vi "Replication and Deployment Utility.vi"() -> ()   [LabVIEW 2016]
uses:
  subVIs/TypeDefs/rad_State Data.ctl
  subVIs/Targets/TypeDefs/rad_Targets Settings.ctl
  subVIs/Targets/TypeDefs/rad_Target Information.ctl
  subVIs/Targets/TypeDefs/rad_Target Network Settings.ctl
  subVIs/App Images/TypeDefs/rad_App Images Settings.ctl
  subVIs/App Images/TypeDefs/rad_AppImage Information.ctl
  subVIs/App Images/TypeDefs/rad_Application Image Properties.ctl
  subVIs/App Images/TypeDefs/rad_FPGA Properties.ctl
  subVIs/App Images/TypeDefs/rad_FPGA Flash Properties.ctl
  subVIs/Util/Controls/Exit Button.ctl
  subVIs/Util/Controls/Retrieve Button.ctl
  subVIs/Util/Controls/Refresh Button.ctl
  subVIs/Util/Controls/Configure Button.ctl
  subVIs/Util/Controls/Deploy Button.ctl
  subVIs/Util/Controls/Select All Button.ctl
  subVIs/Util/Controls/Add Target Button.ctl
  subVIs/Util/Controls/Compare Button.ctl
  subVIs/Util/FP Control/FP Control Functions.ctl
  <vilib>/Utility/miscctls.llb/LVRowAndColumnUnsignedTypeDef.ctl
  subVIs/RT Image Compare/TypeDefs/rad_Comparison Modes.ctl
  subVIs/rad_Globals.vi
  <vilib>/nisyscfg/Close (System).vi
  <vilib>/nisyscfg/nisyscfg.lvlib
  <resource>/objmgr/nisysapi.rc
panel:
  in  "Targets Settings":bool
  in  "Refresh Targets":T1
  in  "Target List":i32[](listbox)=[0]
  in  "Add Target":T2
  in  "Select All":T3
  in  "Configure Targets":T4
  in  "Compare":T5
  in  "Deploy":T6
  in  "Retrieve":T7
  in  "State":T8 {"Targets Information"."Primary NIC"."IP Address Request Mode" items=["Static"=1, "DHCP/Link-Local"=2, "Link-Local Only"=4, "DHCP Only"=8]}
  in  "App Images Settings":bool
  in  "Refresh Apps":T1
  in  "Exit":T17
  in  "App Images List":i32(listbox)=6
  in  "Configure App":T4
  # "Deployment Targets"
  # "Application Images"
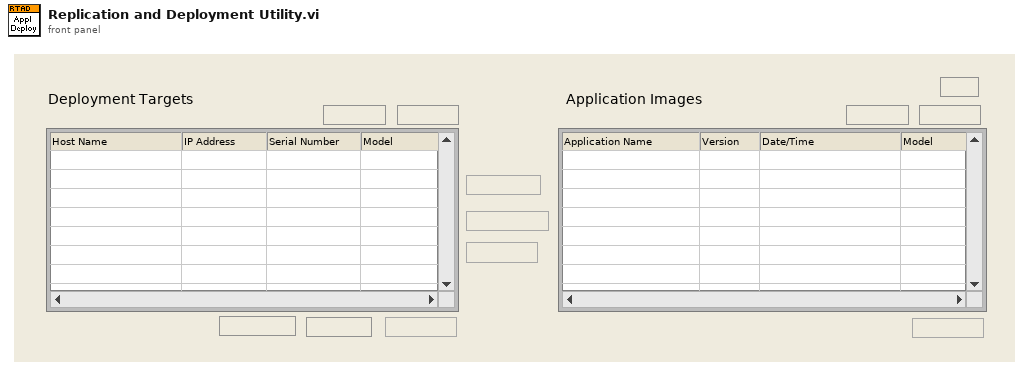
[diagram p1: front panel]
types:
  T1 = typedef "Refresh Button.ctl" = bool
  T2 = typedef "Add Target Button.ctl" = bool
  T3 = typedef "Select All Button.ctl" = bool
  T4 = typedef "Configure Button.ctl" = bool
  T5 = typedef "Compare Button.ctl" = bool
  T6 = typedef "Deploy Button.ctl" = bool
  T7 = typedef "Retrieve Button.ctl" = bool
  T8 = typedef "rad_State Data.ctl" = cluster{"Targets Settings":T9, "Targets Information":T10[], "App Images Settings":T12, "App Images Information":T13[], "Filtered Targets":i32[], "AppMode":string, "Configuration File Path":path, "Permissions":cluster{"Retrieve AppImgs":bool}, "User Added Targets":string[]}
  T9 = typedef "rad_Targets Settings.ctl" = cluster{"Target Types":string[], "Reduce Discovery Timeout":bool}
  T10 = typedef "rad_Target Information.ctl" = cluster{"Hostname":string, "Serial number":string, "Product name":string, "Product code":i32, "System status":string, "Credential type":enum16{"None/Unlocked", "FTP Password", "NIAuth Credentials"}, "User added?":bool, "Primary NIC":T11}
  T11 = typedef "rad_Target Network Settings.ctl" = cluster{"MAC address":string, "IP Address Request Mode":i32, "IP address":string, "Subnet mask":string, "Gateway":string, "DNS server":string}
  T12 = typedef "rad_App Images Settings.ctl" = cluster{"App Images Folder":path, "App Images Temp Folder":path, "CurrentVersion":string}
  T13 = typedef "rad_AppImage Information.ctl" = cluster{"AppImage Properties":T14, "AppImage Path":path}
  T14 = typedef "rad_Application Image Properties.ctl" = cluster{"Name":string, "Version":string, "Time":timestamp, "Description":string, "Key":string, "Chassis":string, "FPGA Properties":T15, "Model":string, "Retrieve":string[], "Deploy":string[], "Installed Software":string[]}
  T15 = typedef "rad_FPGA Properties.ctl" = T16[]
  T16 = typedef "rad_FPGA Flash Properties.ctl" = cluster{"Resource Name":string, "Path":path}
  T17 = typedef "Exit Button.ctl" = bool
  T18 = typedef "LVPoint32TypeDef.ctl" = cluster{"Horizontal":i32, "Vertical":i32}
  T19 = typedef "LVRowAndColumnTypeDef.ctl" = cluster{"Row":i32, "Column":i32}
  T20 = typedef "FP Control Functions.ctl" = enum16{"Open", "Close", "Bring To Front", "Center"}
  T21 = typedef "LVRowAndColumnUnsignedTypeDef.ctl" = cluster{"Row":u32, "Column":u32}
  T22 = typedef "rad_Comparison Modes.ctl" = enum32{"Compare Local Image With Controller", "Compare Two Local Images"}
  T23 = enum8{"Enabled", "Disabled", "Disabled and Grayed Out"}
  T24 = enum32{"invalid app kind", "Development System", "Run Time System", "Student Edition", "Embedded LabVIEW", "Evaluation", "Custom"}
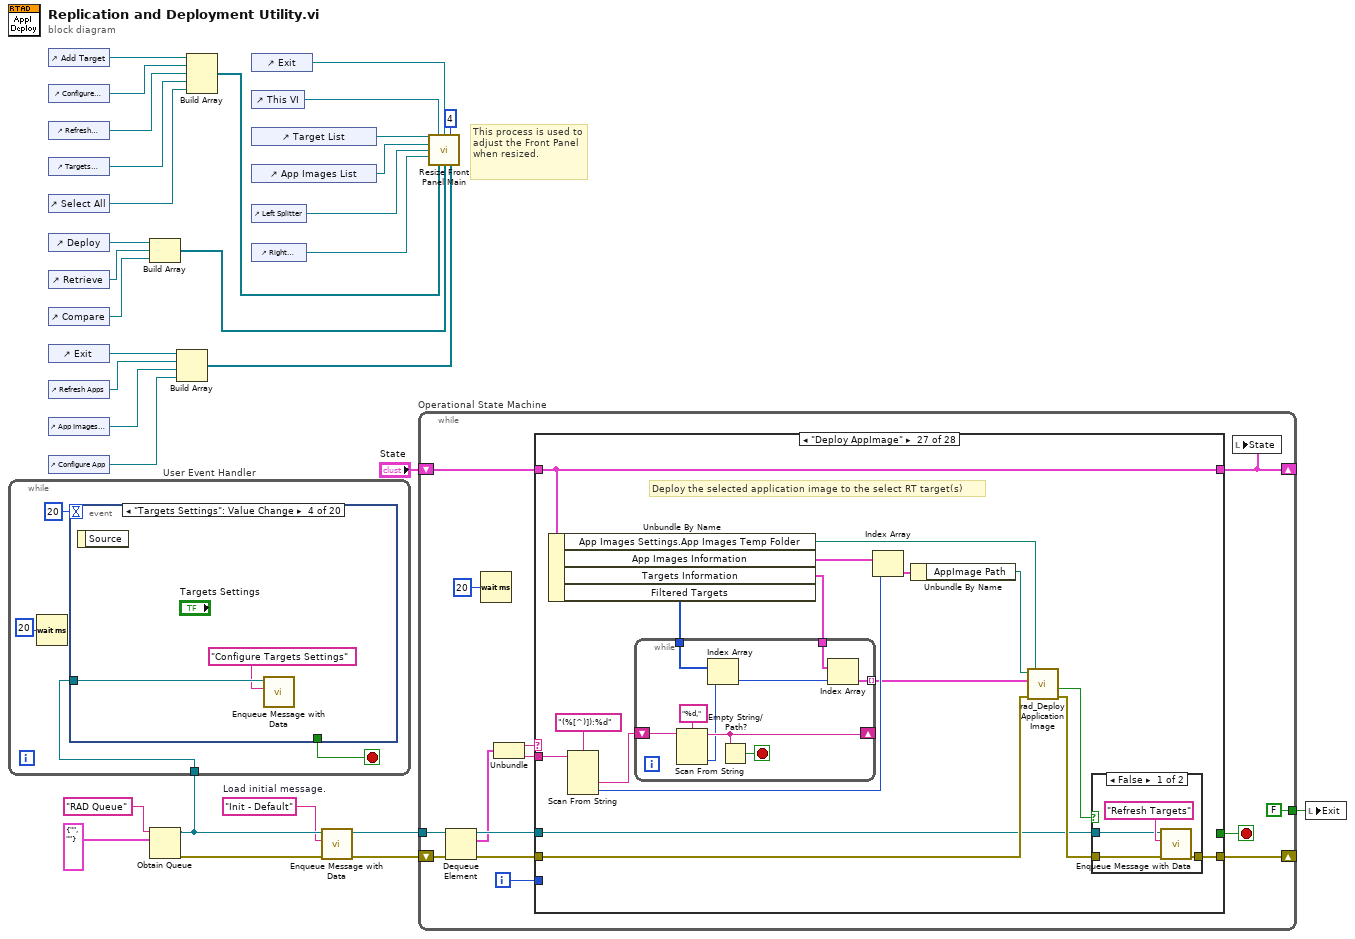
[diagram p0: block diagram]
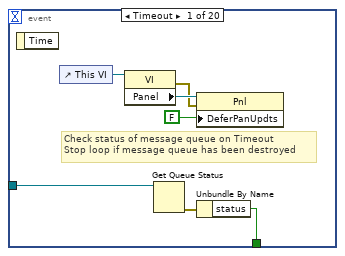
[diagram p2: hidden frame]
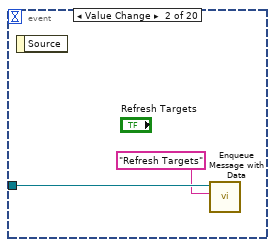
[diagram p3: hidden frame]
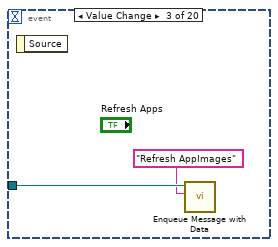
[diagram p4: hidden frame]
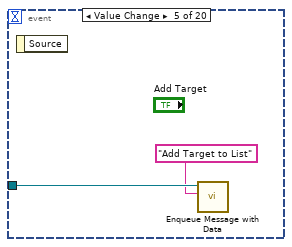
[diagram p5: hidden frame]
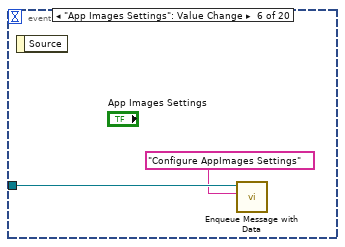
[diagram p6: hidden frame]
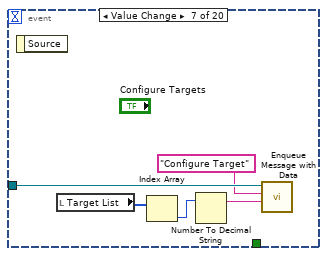
[diagram p7: hidden frame]
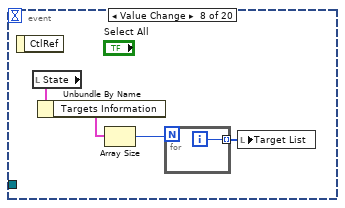
[diagram p8: hidden frame]
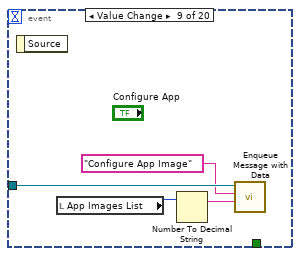
[diagram p9: hidden frame]
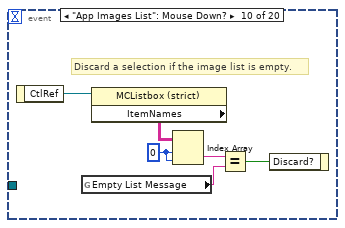
[diagram p10: hidden frame]
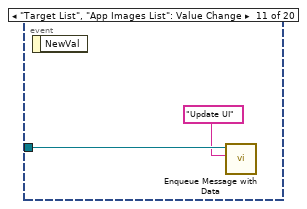
[diagram p11: hidden frame]
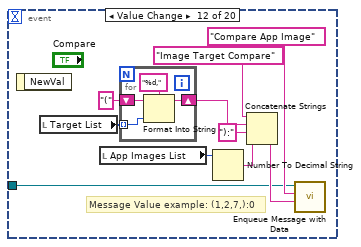
[diagram p12: hidden frame]
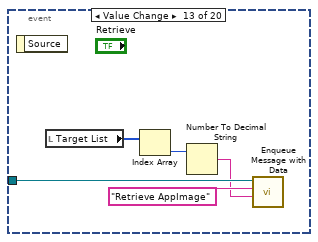
[diagram p13: hidden frame]
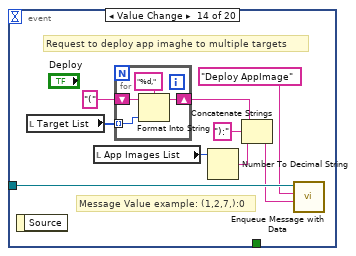
[diagram p14: hidden frame]
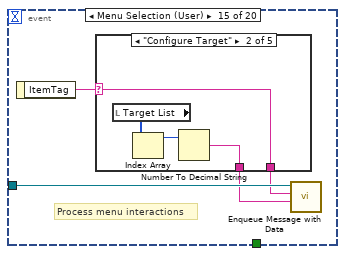
[diagram p15: hidden frame]
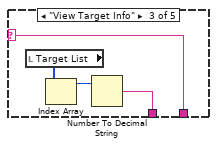
[diagram p17: hidden frame]
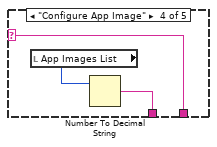
[diagram p18: hidden frame]
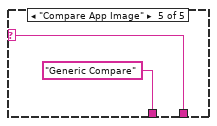
[diagram p19: hidden frame]
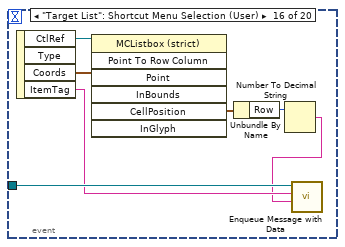
[diagram p20: hidden frame]
diagram:
  w1 = "Init - Default"  # Load initial message.
  # "This process is used to adjust the Front Panel when resized."
  n1 = control-ref of="Add Target"() -> (w22:refnum<vi>)
  n2 = control-ref of="Configure Targets"() -> (w21:refnum<vi>)
  n3 = control-ref of="Refresh Targets"() -> (w20:refnum<vi>)
  n4 = control-ref of="Targets Settings"() -> (w19:refnum<vi>)
  n5 = control-ref of="Select All"() -> (w18:refnum<vi>)
  n6 = control-ref of="Deploy"() -> (w16:refnum<vi>)
  n7 = control-ref of="Retrieve"() -> (w15:refnum<vi>)
  n8 = control-ref of="Compare"() -> (w14:refnum<vi>)
  n9 = control-ref of="Exit"() -> (w12:refnum<vi>)
  n10 = control-ref of="Refresh Apps"() -> (w11:refnum<vi>)
  n11 = control-ref of="App Images Settings"() -> (w10:refnum<vi>)
  n12 = control-ref of="Configure App"() -> (w9:refnum<vi>)
  n13 = Build Array(w16, w15, w14) -> (w13:refnum<vi>[])
  n14 = Obtain Queue(name (unnamed)="RAD Queue" ("message queue name"), element data type=cluster{string, string} {"", ""}) -> (queue out=w6:refnum<queue>, error out=w4:errorcluster)  [unwired: 3 in, 1 out]
  n15 = while "User Event Handler" {
    tunnel: w6 -> [w33]
    stop <- w34 stop-if-true
    n16 = Wait (ms)(milliseconds to wait=u32 20) -> ()  [unwired: 1 out]
    n17 = event shown="[3] \"Targets Settings\": Value Change" {
      selector: _ -> [_ _ _ _ _ _ _ _ _ _ _ _ _ _ _ _ _ _ _ _]
      dyn-events: _ -> [_ _ _ _ _ _ _ _ _ _ _ _ _ _ _ _ _ _ _ _]
      timeout: 20 -> [_ _ _ _ _ _ _ _ _ _ _ _ _ _ _ _ _ _ _ _]
      tunnel: [w40 _ _ _ _ _ _ _ _ _ _ _ _ _ _ _ _ _ TRUE ("Discard?") w156] -> w34
      tunnel: w33 -> [w42 w44 w46 w48 w50 w52 w55 _ w65 _ w74 w77 w91 w96 w109 w127 _ w146 w152 w155]
      event Timeout {
        # "Check status of message queue on Timeout\nStop loop if message queue has been destroyed"
        n18 = event-data() -> ()  [unwired: 2 out]
        n19 = control-ref of="This VI"() -> (w36:refnum<vi>)
        n20 = property class="VI"(reference=w36) -> (error out=w37:errorcluster, "Panel"=w39:refnum<vi>)  [unwired: 1 in, 1 out]
        n21 = Get Queue Status(queue=w42) -> (error out=w41:errorcluster)  [unwired: 1 in, 8 out]
        n22 = property class="Pnl"(reference=w39, error in=w37, "DeferPanUpdts"=FALSE ("Defer Panel Updates")) -> ()  [unwired: 2 out]
        n23 = Unbundle By Name(w41) -> ("status"=w40:bool)
      }
      event Value Change {
        n24 = event-data() -> ()  [unwired: 2 out]
        n25 = call "Enqueue Message with Data.vi"("message ID"="Refresh Targets", "queue in"=w44) -> ()  [unwired: 8 in, 2 out]
      }
      event Value Change {
        n26 = event-data() -> ()  [unwired: 2 out]
        n27 = call "Enqueue Message with Data.vi"("message ID"="Refresh AppImages", "queue in"=w46) -> ()  [unwired: 8 in, 2 out]
      }
      event "Targets Settings": Value Change {
        n28 = event-data() -> ()  [unwired: 2 out]
        n29 = call "Enqueue Message with Data.vi"("message ID"="Configure Targets Settings", "queue in"=w48) -> ()  [unwired: 8 in, 2 out]
      }
      event Value Change {
        n30 = event-data() -> ()  [unwired: 2 out]
        n31 = call "Enqueue Message with Data.vi"("message ID"="Add Target to List" ("Message Name"), "queue in"=w50) -> ()  [unwired: 8 in, 2 out]
      }
      event "App Images Settings": Value Change {
        n32 = event-data() -> ()  [unwired: 2 out]
        n33 = call "Enqueue Message with Data.vi"("message ID"="Configure AppImages Settings", "queue in"=w52) -> ()  [unwired: 8 in, 2 out]
      }
      event Value Change {
        n34 = event-data() -> ()  [unwired: 2 out]
        n35 = local read "Target List"() -> (w56:i32[])
        n36 = Index Array(array=w56) -> (element=w57:i32)  [unwired: 1 in]
        n37 = Number To Decimal String(number=w57) -> (decimal integer string=w53:string)  [unwired: 1 out]
        n38 = call "Enqueue Message with Data.vi"("extra data"=w53, "message ID"="Configure Target", "queue in"=w55) -> ()  [unwired: 7 in, 2 out]
      }
      event Value Change {
        n39 = event-data() -> ()  [unwired: 2 out]
        n40 = local read "State"() -> (w60:T8)
        n41 = Unbundle By Name(w60) -> ("Targets Information"=w59:T10[])
        n42 = Array Size(array=w59) -> (size(s)=w58:i32)
        n43 = for {
          N: w58 -> [_]
          tunnel: [w62] -> w61 mode=indexing
          i -> [w62]
        }
        n44 = local write "Target List"(w61) -> ()
      }
      event Value Change {
        n45 = event-data() -> ()  [unwired: 2 out]
        n46 = local read "App Images List"() -> (w66:i32)
        n47 = Number To Decimal String(number=w66) -> (decimal integer string=w63:string)  [unwired: 1 out]
        n48 = call "Enqueue Message with Data.vi"("extra data"=w63, "message ID"="Configure App Image", "queue in"=w65) -> ()  [unwired: 7 in, 2 out]
      }
      event "App Images List": Mouse Down? {
        w70 = 0 ("index (row)")
        # "Discard a selection if the image list is empty."
        n49 = event-data() -> ("CtlRef"=w72:refnum<vi>)  [unwired: 1 out]
        n50 = global read "rad_Globals.vi" "Empty List Message"() -> (w68:string)
        n51 = property class="MCListbox (strict)"(reference=w72) -> ("ItemNames"=w71:string[][])  [unwired: 1 in, 2 out]
        n52 = Index Array(array=w71, index (row)=w70, index (col)=w70) -> (element=w69:string)
        n53 = Equal?(x=w69, y=w68) -> (x = y?=w67:bool)
        n54 = event-data("Discard?"=w67) -> ()  [unwired: 1 in, 1 out]
      }
      event "Target List", "App Images List": Value Change {
        n55 = event-data() -> ()  [unwired: 2 out]
        n56 = call "Enqueue Message with Data.vi"("message ID"="Update UI" ("Message"), "queue in"=w74) -> ()  [unwired: 8 in, 2 out]
      }
      event Value Change {
        # "Message Value example: (1,2,7,):0"
        n57 = event-data() -> ()  [unwired: 2 out]
        n58 = local read "Target List"() -> (w81:i32[])
        n59 = local read "App Images List"() -> (w80:i32)
        n60 = for {
          shift-right: [w88] -> w82
          shift-left: "(" -> [w86]
          tunnel: w81 -> [w87] mode=indexing
          n61 = Format Into String(format string="%d,", initial string=w86, w87) -> (resulting string=w88:string)  [unwired: 1 in, 1 out]
        }
        n62 = Number To Decimal String(number=w80) -> (decimal integer string=w79:string)  [unwired: 1 out]
        n63 = Concatenate Strings("Image Target Compare" ("string"), w82, "):" ("string"), w79) -> (w84:string)
        n64 = call "Enqueue Message with Data.vi"("extra data"=w84, "message ID"="Compare App Image", "queue in"=w77) -> ()  [unwired: 7 in, 2 out]
      }
      event Value Change {
        n65 = event-data() -> ()  [unwired: 2 out]
        n66 = local read "Target List"() -> (w92:i32[])
        n67 = Index Array(array=w92) -> (element=w93:i32)  [unwired: 1 in]
        n68 = Number To Decimal String(number=w93) -> (decimal integer string=w89:string)  [unwired: 1 out]
        n69 = call "Enqueue Message with Data.vi"("extra data"=w89, "message ID"="Retrieve AppImage", "queue in"=w91) -> ()  [unwired: 7 in, 2 out]
      }
      event Value Change {
        # "Request to deploy app imaghe to multiple targets"
        # "Message Value example: (1,2,7,):0"
        n70 = event-data() -> ()  [unwired: 2 out]
        n71 = local read "Target List"() -> (w98:i32[])
        n72 = local read "App Images List"() -> (w100:i32)
        n73 = for {
          shift-right: [w106] -> w97
          shift-left: "(" -> [w104]
          tunnel: w98 -> [w105] mode=indexing
          n74 = Format Into String(format string="%d,", initial string=w104, w105) -> (resulting string=w106:string)  [unwired: 1 in, 1 out]
        }
        n75 = Number To Decimal String(number=w100) -> (decimal integer string=w101:string)  [unwired: 1 out]
        n76 = Concatenate Strings(w97, "):" ("string"), w101) -> (w94:string)
        n77 = call "Enqueue Message with Data.vi"("extra data"=w94, "message ID"="Deploy AppImage", "queue in"=w96) -> ()  [unwired: 7 in, 2 out]
      }
      event Menu Selection (User) {
        # "Process menu interactions"
        n78 = event-data() -> ("ItemTag"=w110:string)  [unwired: 1 out]
        n79 = case shown="\"Configure Target\"" w110 {
          selector: w110 -> [w111 w113 w117 w121 w123]
          tunnel: [w111 w113 w117 w121 w123] -> w108
          tunnel: [_ w112 w116 w120 "Generic Compare"] -> w107
          frame Default {
          }
          frame "Configure Target" {
            n80 = local read "Target List"() -> (w115:i32[])
            n81 = Index Array(array=w115) -> (element=w114:i32)  [unwired: 1 in]
            n82 = Number To Decimal String(number=w114) -> (decimal integer string=w112:string)  [unwired: 1 out]
          }
          frame "View Target Info" {
            n83 = local read "Target List"() -> (w119:i32[])
            n84 = Index Array(array=w119) -> (element=w118:i32)  [unwired: 1 in]
            n85 = Number To Decimal String(number=w118) -> (decimal integer string=w116:string)  [unwired: 1 out]
          }
          frame "Configure App Image" {
            n86 = local read "App Images List"() -> (w122:i32)
            n87 = Number To Decimal String(number=w122) -> (decimal integer string=w120:string)  [unwired: 1 out]
          }
          frame "Compare App Image" {
          }
        }
        n88 = call "Enqueue Message with Data.vi"("extra data"=w107, "message ID"=w108, "queue in"=w109) -> ()  [unwired: 7 in, 2 out]
      }
      event "Target List": Shortcut Menu Selection (User) {
        n89 = event-data() -> ("CtlRef"=w129:refnum<vi>, "Coords"=w128:T18, "ItemTag"=w126:string)  [unwired: 2 out]
        n90 = invoke class="MCListbox (strict)" method="Point To Row Column"(reference=w129, "Point"=w128) -> ("CellPosition"=w131:T19)  [unwired: 5 in, 6 out]
        n91 = Unbundle By Name(w131) -> ("Row"=w130:i32)
        n92 = Number To Decimal String(number=w130) -> (decimal integer string=w125:string)  [unwired: 1 out]
        n93 = call "Enqueue Message with Data.vi"("extra data"=w125, "message ID"=w126, "queue in"=w127) -> ()  [unwired: 7 in, 2 out]
      }
      event "App Images List": Shortcut Menu Activation? {
        n94 = event-data() -> ("MenuRef"=w133:refnum<k9>)  [unwired: 1 out]
        n95 = global read "rad_Globals.vi" "Manager Permissions"() -> (w132:bool)
        n96 = case shown="False" w132 {
          tunnel: w133 -> [w138 _]
          tunnel: [w135 _] -> _
          frame False {
            w134 = string[] ["View App Image Info"] ("item names")
            n97 = Delete Menu Items(9:w138) -> (0:w136:errorcluster, 3:w137:refnum<k9>)  [unwired: 3 in]
            n98 = Insert Menu Items(6:w136, 7:w134, 8:w134, 9:w137) -> (0:w135:errorcluster)  [unwired: 2 in, 2 out]
          }
          frame True {
          }
        }
        n99 = event-data() -> ()  [unwired: 2 in, 1 out]
      }
      event "App Images List": Shortcut Menu Selection (User) {
        n100 = event-data() -> ("CtlRef"=w148:refnum<vi>, "Coords"=w147:T18, "ItemTag"=w139:string)  [unwired: 1 out]
        n101 = Equal?(x=w139, y="Compare App Image") -> (x = y?=w144:bool)
        n102 = invoke class="MCListbox (strict)" method="Point To Row Column"(reference=w148, "Point"=w147) -> ("CellPosition"=w150:T19)  [unwired: 5 in, 6 out]
        n103 = Unbundle By Name(w150) -> ("Row"=w149:i32)
        n104 = Number To Decimal String(number=w149) -> (decimal integer string=w141:string)  [unwired: 1 out]
        n105 = Concatenate Strings("Only Image Selected(" ("string"), w141) -> (w143:string)
        n106 = Select(t=w143, s=w144, f=w141) -> (s? t:f=w140:string)
        n107 = call "Enqueue Message with Data.vi"("extra data"=w140, "message ID"=w139, "queue in"=w146) -> ()  [unwired: 7 in, 2 out]
      }
      event Value Change {
        n108 = event-data() -> ()  [unwired: 2 out]
        n109 = call "Enqueue Message with Data.vi"("message ID"="Exit", "queue in"=w152) -> ()  [unwired: 8 in, 2 out]
      }
      event Panel Close? {
        w156 = TRUE ("Discard?")
        # "Intercepts the upper right close panel\noperation to allow a smooth shutdown\nas opposed to immediately killing the app."
        n110 = event-data() -> ()  [unwired: 2 out]
        n111 = call "Enqueue Message with Data.vi"("message ID"="Exit", "queue in"=w155) -> ()  [unwired: 8 in, 2 out]
        n112 = event-data("Discard?"=w156) -> ()  [unwired: 1 in, 1 out]
      }
    }
  }
  n113 = Build Array(w12, w11, w10, w9) -> (w8:refnum<vi>[])
  n114 = Build Array(w22, w21, w20, w19, w18) -> (w17:refnum<vi>[])
  n115 = control-ref of="Exit"() -> (w28:refnum<vi>)
  n116 = control-ref of="This VI"() -> (w27:refnum<vi>)
  n117 = control-ref of="Target List"() -> (w26:refnum<vi>)
  n118 = control-ref of="App Images List"() -> (w25:refnum<vi>)
  n119 = control-ref of="Left Splitter"() -> (w24:refnum<vi>)
  n120 = control-ref of="Right Splitter"() -> (w23:refnum<vi>)
  n121 = call "Enqueue Message with Data.vi"("error in (no error)"=w4, "message ID"=w1, "queue in"=w6) -> ("error out"=w3:errorcluster, "queue out"=w5:refnum<queue>)  [unwired: 7 in]
  n122 = while "Operational State Machine" {
    shift-left: w3 -> [w162]
    shift-right: [w163] -> _
    tunnel: w5 -> [w167]
    shift-left: "State" -> [w170]
    shift-right: [w164] -> _
    tunnel: [T17 FALSE ("Exit")] -> w7
    i -> [w166]
    stop <- w160 stop-if-true
    n123 = Dequeue Element(queue=w167, error in (no error)=w162) -> (queue out=w169:refnum<queue>, element=w165:cluster{string, string}, error out=w168:errorcluster)  [unwired: 1 in, 1 out]
    n124 = Wait (ms)(milliseconds to wait=u32 20) -> ()  [unwired: 1 out]
    n125 = Unbundle(w165) -> (w159:string, w158:string)
    n126 = case shown="\"Deploy AppImage\"" w159 {
      tunnel: [w172 w174 w188 w216 w237 w258 w289 w304 w306 w310 w316 w328 w336 w352 w374 w390 w406 w419 w430 w432 w453 w468 w480 w488 w557 w572 w604 w620] -> w164
      tunnel: w170 -> [w172 w174 w192 w215 w238 w254 w289 w304 w306 w310 w316 w328 w337 w353 w375 w391 w406 w424 w430 w436 w454 w467 w480 w488 w557 w573 w604 w620]
      tunnel: w169 -> [_ _ w176 w198 _ w250 _ _ _ _ w323 _ w334 w348 w373 w389 _ w418 _ w434 w447 w470 _ _ w544 w576 w589 w621]
      tunnel: w168 -> [w171 w173 w181 w197 w236 w252 w286 w305 w307 w309 w322 w327 w333 w350 w369 w388 w399 w417 w429 w433 w449 w469 w481 w487 w546 w579 w592 w625]
      tunnel: w166 -> [_ _ _ _ _ _ _ _ _ _ _ _ _ _ _ _ _ _ _ _ _ _ _ _ _ _ _ _]
      tunnel: w158 -> [_ _ _ _ _ _ _ _ _ _ _ _ _ _ w383 _ w404 w428 _ _ w457 _ w477 w484 w555 w581 w603 _]
      tunnel: [w171 w173 w175 w200 w236 w251 w270 w305 w307 errorcluster {"status"=FALSE, "code"=0, "source"=""} ("error out") w317 w327 w335 w349 w371 w385 w399 w416 w429 w435 w448 w464 w481 w482 w545 w577 w591 w622] -> w163
      tunnel: [_ _ _ _ _ _ _ _ _ _ TRUE _ _ _ _ _ _ _ _ _ _ _ _ _ _ _ _ _] -> w160
      frame "Missing Message Handler", Default {
      }
      frame "**** General Application Messages ****" {
      }
      frame "Init - Default" {
        w182 = T21 {"Row"=0, "Column"=0} ("Top Left Visible Cell")
        w184 = string[][] [] ("Item Names")
        w191 = u8 2 ("Disabled")
        # "Initialize the UI"
        # "Application Folder"
        # "Default AppImages folder"
        n127 = call "Util_App Application Directory.vi"() -> ("Application Directory"=w187:path)  [unwired: 11 out]
        n128 = call "Enqueue Message with Data.vi"("error in (no error)"=w181, "message ID"="Init - Load Config", "queue in"=w176) -> ("error out"=w180:errorcluster, "queue out"=w179:refnum<queue>)  [unwired: 7 in]
        n129 = local write "App Images List"(-1 ("App Images List")) -> ()
        n130 = local write "Target List"(i32[] [] ("Target List")) -> ()
        n131 = Build Path(base path=w187, name or relative path="appimages") -> (appended path=w193:path)
        n132 = Build Path(base path=w187, name or relative path="rad_config.ini" ("Config File Name")) -> (appended path=w185:path)
        n133 = call "Enqueue Message with Data.vi"("error in (no error)"=w180, "message ID"="Init - Configure Settings", "queue in"=w179) -> ("error out"=w175:errorcluster)  [unwired: 7 in, 1 out]
        n134 = property on="Configure App" class="Bool"("Disabled"=w191) -> ()  [unwired: 2 in, 2 out]
        n135 = property on="Configure Targets" class="Bool"("Disabled"=w191) -> ()  [unwired: 2 in, 2 out]
        n136 = Bundle By Name(cluster=w192, "App Images Settings.App Images Folder"=w193, "Configuration File Path"=w185) -> (w188:T8)
        n137 = property on="Target List" class="MCListbox (strict)"("ItemNames"=w184, "TopLeft"=w182) -> ()  [unwired: 2 in, 2 out]
        n138 = property on="App Images List" class="MCListbox (strict)"("ItemNames"=w184, "TopLeft"=w182) -> ()  [unwired: 2 in, 2 out]
        n139 = call "Util_FP Control.vi"("Function"=FP_Control_Functions."Center") -> ()  [unwired: 10 in, 1 out]
      }
      frame "Init - Load Config" {
        n140 = call "rad_Load Config.vi"("error in (no error"=w197, "State in"=w215) -> ("error out"=w195:errorcluster, "State out"=w216:T8)  [unwired: 1 in, 7 out]
        n141 = call <vilib>:"Initialize Session.vi"("error in (no error)"=w195) -> ("error out"=w203:errorcluster, "Session out"=w204:refnum<k21>)  [unwired: 9 in]
        n142 = property class="System Session"(reference=w204, error in=w203) -> (reference out=w205:refnum<k21>, error out=w202:errorcluster, "InstalledVer"=w201:string)
        n143 = Scan From String(format string="%d.%d.%d", input string=w201) -> (output 1=w213:i32, output 2=w210:i32, output 3=w207:i32)  [unwired: 5 in, 3 out]
        n144 = call-poly <vilib>:"Close.vi"("error in (no error)"=w202, "Session in"=w205) -> ("error out"=w199:errorcluster)  [unwired: 9 in]
        n145 = Multiply(x=10, y=w210) -> (x*y=w208:i32)
        n146 = Multiply(x=100, y=w213) -> (x*y=w209:i32)
        n147 = Compound Arithmetic op=ADD(w209, w208, w207) -> (w206:i32)
        n148 = case shown="Default" w206 {
          tunnel: [w227 TRUE ("T button?")] -> w196
          tunnel: w199 -> [_ _]
          frame Default {
            n149 = Two Button Dialog(message="RAD requires newer functionality\nthan the software you have installed.\nPlease update to NI System Configuration\nversion 14.0 or higher.", 1:"Exit" ("F button name (\"Cancel\")"), 2:"Continue" ("T button name (\"OK\")")) -> (T button?=w227:bool)
          }
          frame 1400.. {
            # "RAD 14.0 has been fully tested\nwith NI System Configuration 14.0.\nFuture versions should work fine too."
          }
        }
        n150 = case shown="True" w196 {
          tunnel: w195 -> [w218 w225]
          tunnel: [w219 w220] -> w200
          tunnel: w198 -> [_ w224]
          frame False {
            n151 = property on="Exit" class="Bool (strict)"(error in=w218, "Val(Sgnl)"=T17 TRUE ("Value (Signaling)")) -> (error out=w219:errorcluster)  [unwired: 1 in, 1 out]
          }
          frame True {
            n152 = call "Enqueue Message with Data.vi"("error in (no error)"=w225, "message ID"="Refresh Targets", "queue in"=w224) -> ("error out"=w221:errorcluster, "queue out"=w222:refnum<queue>)  [unwired: 7 in]
            n153 = call "Enqueue Message with Data.vi"("error in (no error)"=w221, "message ID"="Refresh AppImages", "queue in"=w222) -> ("error out"=w220:errorcluster)  [unwired: 7 in, 1 out]
          }
        }
      }
      frame "Init - Configure Settings" {
        # "The temp folder should always be writable."
        # "Set permissions and update UI based on application\nmode. Disable or hide controls not appropriate\nfor current application mode."
        # "Apply configuration settings from config file"
        n154 = Unbundle By Name(w238) -> ("AppMode"=w239:string)
        n155 = case shown="\"Manager\"" w239 {
          tunnel: [TRUE ("Visible") FALSE ("Visible")] -> w235
          frame "Manager" {
          }
          frame Default {
          }
        }
        n156 = call <vilib>:"Generate Temporary File Path.vi"("Temporary File Extension (tmp)"="rad") -> ("Unique Temporary File Path"=w232:path)  [unwired: 9 in, 1 out]
        n157 = property on="Retrieve" class="Bool"("Visible"=w235) -> ()  [unwired: 2 in, 2 out]
        n158 = property on="Configure App" class="Bool"("Visible"=w235) -> ()  [unwired: 2 in, 2 out]
        n159 = Bundle By Name(cluster=w238, "App Images Settings.App Images Temp Folder"=w232, "Permissions.Retrieve AppImgs"=w235) -> (w237:T8)
        n160 = global write "rad_Globals.vi" "Manager Permissions"(w235) -> ()
        n161 = global write "rad_Globals.vi" "ShownImageVersionDialog"(FALSE ("ShownNewerVersionDialog")) -> ()
      }
      frame "Update UI" {
        # "Scroll the lists to the top if no item is selected."
        # "Display target and app images based on settings\nfor each of these tables"
        n162 = Unbundle By Name(w254) -> ("Targets Information"=w261:T10[], "Targets Settings.Target Types"=w253:string[], "App Images Information"=w255:T13[])
        n163 = call "rad_Format Application Images Information.vi"("App Images Information"=w255) -> ("App Images Information"=w256:string[][])  [unwired: 10 out]
        n164 = call "rad_FilterTargets.vi"("Target Types"=w253, "Targets Information"=w261) -> ("Filtered Targets"=w259:i32[], "Targets Information"=w260:T10[])  [unwired: 8 out]
        n165 = Bundle By Name(cluster=w254, "Filtered Targets"=w259) -> (w258:T8)
        n166 = call "rad_Format Target Information.vi"("Targets Information"=w260) -> ("Targets Information"=w257:string[][])  [unwired: 10 out]
        n167 = property on="App Images List" class="MCListbox (strict)"("ItemNames"=w256) -> (error out=w247:errorcluster)  [unwired: 2 in, 1 out]
        n168 = property on="Target List" class="MCListbox (strict)"("ItemNames"=w257) -> (error out=w248:errorcluster)  [unwired: 2 in, 1 out]
        n169 = flat-sequence {
          tunnel: w248 -> [_]
          tunnel: w247 -> [_]
          tunnel: ["App Images List"] -> w245
          tunnel: [w265] -> w246
          tunnel: [-1 ("y")] -> w243
          frame #0 {
            n170 = Array Size(array="Target List") -> (size(s)=w265:i32)
          }
        }
        n171 = Equal?(x=w245, y=w243) -> (x = y?=w242:bool)
        n172 = Equal To 0?(x=w246) -> (x = 0?=w244:bool)
        n173 = call "Enqueue Message with Data.vi"("error in (no error)"=w252, "message ID"="Update Buttons and Menus" ("Message Name"), "queue in"=w250) -> ("error out"=w251:errorcluster)  [unwired: 7 in, 1 out]
        n174 = case shown="True" w242 {
          frame False {
          }
          frame True {
            n175 = property on="App Images List" class="MCListbox (strict)"("TopLeft"=T21 {"Row"=0, "Column"=0} ("Top Left Visible Cell")) -> ()  [unwired: 2 in, 2 out]
          }
        }
        n176 = case shown="True" w244 {
          frame False {
          }
          frame True {
            n177 = property on="Target List" class="MCListbox (strict)"("TopLeft"=T21 {"Row"=0, "Column"=0} ("Top Left Visible Cell")) -> ()  [unwired: 2 in, 2 out]
          }
        }
      }
      frame "Update Buttons and Menus" {
        w274 = T23."Disabled and Grayed Out" ("Disabled")
        w275 = T23."Enabled" ("Disabled")
        # "Enable and disable buttons and \nenu items based on selections\nin both tables"
        n178 = local read "App Images List"() -> (w287:i32)
        n179 = local read "Target List"() -> (w288:i32[])
        n180 = Unbundle By Name(w289) -> ("Permissions.Retrieve AppImgs"=w268:bool)
        n181 = call "rad_Button and Menu Status.vi"("Manager Permissions"=w268, "App Image List"=w287, "Target List"=w288) -> ("Retrieve AppImage"=w278:bool, "Deploy AppImage"=w280:bool, "View Target Info"=w285:bool, "Configure App Image"=w282:bool, "Compare"=w276:bool, "Configure Target"=w284:bool)  [unwired: 3 in]
        n182 = Current VI's Menubar() -> (w290:refnum<k9>)
        n183 = Set Menu Item Info(7:"Configure Target" ("item tag"), 8:w286, 9:w284, 11:w290) -> (0:w292:errorcluster, 3:w294:refnum<k9>)  [unwired: 3 out]
        n184 = Select(t=w275, s=w284, f=w274) -> (s? t:f=w283:T23)
        n185 = Select(t=w275, s=w282, f=w274) -> (s? t:f=w281:T23)
        n186 = Select(t=w275, s=w280, f=w274) -> (s? t:f=w279:T23)
        n187 = Select(t=w275, s=w278, f=w274) -> (s? t:f=w277:T23)
        n188 = Select(t=w275, s=w276, f=w274) -> (s? t:f=w273:T23)
        n189 = Set Menu Item Info(7:"Configure App Image" ("item tag"), 8:w292, 9:w282, 11:w294) -> (0:w295:errorcluster, 3:w296:refnum<k9>)  [unwired: 3 out]
        n190 = Set Menu Item Info(7:"View Target Info" ("item tag"), 8:w295, 9:w285, 11:w296) -> (0:w297:errorcluster, 3:w298:refnum<k9>)  [unwired: 3 out]
        n191 = Set Menu Item Info(7:"Deploy AppImage" ("item tag"), 8:w297, 9:w280, 11:w298) -> (0:w299:errorcluster, 3:w300:refnum<k9>)  [unwired: 3 out]
        n192 = property on="Configure Targets" class="Bool"("Disabled"=w283) -> ()  [unwired: 2 in, 2 out]
        n193 = property on="Configure App" class="Bool"("Disabled"=w281) -> ()  [unwired: 2 in, 2 out]
        n194 = property on="Deploy" class="Bool"("Disabled"=w279) -> ()  [unwired: 2 in, 2 out]
        n195 = property on="Retrieve" class="Bool"("Disabled"=w277) -> ()  [unwired: 2 in, 2 out]
        n196 = property on="Compare" class="Bool"("DisabledEnum"=w273) -> ()  [unwired: 2 in, 2 out]
        n197 = Set Menu Item Info(7:"Retrieve AppImage" ("item tag"), 8:w299, 9:w278, 11:w300) -> (0:w271:errorcluster, 3:w272:refnum<k9>)  [unwired: 3 out]
        n198 = Set Menu Item Info(7:"Convert Images" ("item tag"), 8:w271, 9:w268, 11:w272) -> (0:w270:errorcluster)  [unwired: 4 out]
      }
      frame "Status" {
      }
      frame "About" {
        # "Show About dialog"
        n199 = call "rad_About Dialog.vi"() -> ()  [unwired: 12 out]
      }
      frame "Error" {
        # "Display run-time error message\nAdd code to log error if desired"
        n200 = disable-structure shown="TARGET_TYPE==Windows" {
          disable-tunnel: w309 -> [w311 _]
          frame condition #0 (active) {
            n201 = call <vilib>:"Simple Error Handler.vi"("error in (no error)"=w311) -> ()  [unwired: 1 in, 8 out]
          }
          frame condition #1 {
          }
        }
      }
      frame "Exit" {
        # "Store current settings in the application config file"
        # "Close the front panel if the application is running as an EXE"
        n202 = Release Queue(queue=w323, force destroy? (F)=TRUE, error in (no error)=w322) -> (error out=w315:errorcluster)  [unwired: 2 out]
        n203 = Open Application Reference() -> (0:w320:errorcluster, 3:w321:refnum<vi>)  [unwired: 4 in]
        n204 = call "rad_Save Config.vi"("error in (no error"=w315, "State"=w316) -> ("error out"=w314:errorcluster)  [unwired: 1 in, 8 out]
        n205 = property class="App"(reference=w321, error in=w320) -> ("App.Kind"=w319:T24)  [unwired: 2 out]
        n206 = case shown="\"Run Time System\"" w319 {
          frame Default {
          }
          frame "Run Time System" {
            # "Close FP in EXE"
            n207 = Current VI's Path() -> (path=w326:path)
            n208 = Open VI Reference(vi path=w326) -> (vi reference=w325:refnum<vi>, error out=w324:errorcluster)  [unwired: 5 in]
            n209 = invoke class="VI" method="FP.Close"(reference=w325, error in=w324) -> ()  [unwired: 1 in, 3 out]
          }
        }
        n210 = property on="Exit" class="Bool (strict)"(error in=w314, "Val(Sgnl)"=TRUE) -> (error out=w317:errorcluster)  [unwired: 1 in, 1 out]
      }
      frame "**** Target Messages ****" {
      }
      frame "Refresh Targets" {
        # "Refresh list of RT targets on the local subnet.\nShow progress dialog during this process."
        n211 = Unbundle By Name(w337) -> ("Targets Settings.Reduce Discovery Timeout"=w330:bool, "User Added Targets"=w343:string[], "Targets Settings.Target Types"=w329:string[])
        n212 = call "Util_Progress Show Progress Popup.vi"("error in (no error)"=w333, "Title"="Discovering Targets", "Message"="Refreshing target list...") -> ("error out"=w331:errorcluster)  [unwired: 1 in, 7 out]
        n213 = Search 1D Array(1D array=w329, element="User Targets Only") -> (index of element=w340:i32)  [unwired: 1 in]
        n214 = Not Equal?(x=w340, y=-1) -> (x != y?=w338:bool)
        n215 = call "rad_Refresh Target Information.vi"("Reduce Discovery Timeout"=w330, "error in (no error)"=w331, "User Added Targets Only"=w338, "User Added Targets"=w343) -> ("error out"=w332:errorcluster, "Targets Information"=w342:T10[])  [unwired: 6 in]
        n216 = call "Util_Progress Close Progress Popup.vi"("error in (no error)"=w332) -> ()  [unwired: 2 in, 9 out]
        n217 = Bundle By Name(cluster=w337, "Targets Information"=w342) -> (w336:T8)
        n218 = call "Enqueue Message with Data.vi"("error in (no error)"=w332, "message ID"="Update UI", "queue in"=w334) -> ("error out"=w335:errorcluster)  [unwired: 7 in, 1 out]
      }
      frame "Add Target to List" {
        n219 = Unbundle By Name(w353) -> ("User Added Targets"=w355:string[])
        n220 = call "rad_Add Target By IP Dialog.vi"() -> ("Canceled?"=w347:bool, "IP Address"=w354:string)  [unwired: 10 in]
        n221 = case shown="False" w347 {
          tunnel: w355 -> [w363 w368]
          tunnel: w354 -> [w362 _]
          tunnel: [w364 w368] -> w351
          frame False {
            n222 = Search 1D Array(1D array=w363, element=w362) -> (index of element=w367:i32)  [unwired: 1 in]
            n223 = Build Array (concatenate)(w363, w362) -> (w361:string[])
            n224 = Not Equal?(x=w367, y=-1) -> (x != y?=w365:bool)
            n225 = Select(t=w363, s=w365, f=w361) -> (s? t:f=w364:string[])
          }
          frame True {
          }
        }
        n226 = case shown="False" w347 {
          tunnel: w350 -> [w359 w360]
          tunnel: [w358 w360] -> w349
          tunnel: w348 -> [w357 _]
          frame False {
            n227 = call "Enqueue Message with Data.vi"("error in (no error)"=w359, "message ID"="Refresh Targets" ("Message Name"), "queue in"=w357) -> ("error out"=w358:errorcluster)  [unwired: 7 in, 1 out]
          }
          frame True {
          }
        }
        n228 = Bundle By Name(cluster=w353, "User Added Targets"=w351) -> (w352:T8)
      }
      frame "Configure Target" {
        # "Update network settings/configuration of the selected RT target"
        n229 = Unbundle By Name(w375) -> ("Targets Information"=w379:T10[], "Filtered Targets"=w382:i32[])
        n230 = Decimal String To Number(string=w383) -> (number=w381:i32)  [unwired: 3 out]
        n231 = Index Array(array=w382, index=w381) -> (element=w377:i32)
        n232 = Index Array(array=w379, index=w377) -> (element=w380:T10)
        n233 = call "rad_Configure Target Dialog.vi"("Error In"=w369, "Target Information in"=w380) -> ("Error Out"=w370:errorcluster, "Target Information out"=w378:T10)  [unwired: 8 out]
        n234 = Replace Array Subset(array=w379, new element=w378, index=w377) -> (w376:T10[])
        n235 = call <vilib>:"General Error Handler.vi"("error in (no error)"=w370) -> ()  [unwired: 10 in, 5 out]
        n236 = Bundle By Name(cluster=w375, "Targets Information"=w376) -> (w374:T8)
        n237 = call "Enqueue Message with Data.vi"("error in (no error)"=w369, "message ID"="Update UI", "queue in"=w373) -> ("error out"=w371:errorcluster)  [unwired: 7 in, 1 out]
      }
      frame "Configure Targets Settings" {
        # "Update the RT Target settings >> select which types of RT targets to display in the table\nCompactRIO, PXI, FieldPoint, or Other"
        n238 = Unbundle By Name(w391) -> ("Targets Settings"=w386:T9)
        n239 = call "rad_Configure Targets Settings Dialog.vi"("Targets Settings"=w386) -> ("Targets Settings"=w387:T9)  [unwired: 10 out]
        n240 = Equal?(x=w387, y=w386) -> (x = y?=w384:bool)
        n241 = Bundle By Name(cluster=w391, "Targets Settings"=w387) -> (w390:T8)
        n242 = case shown="False" w384 {
          tunnel: w389 -> [w395 _]
          tunnel: w388 -> [w394 w396]
          tunnel: [w393 w396] -> w385
          frame False {
            n243 = call "Enqueue Message with Data.vi"("error in (no error)"=w394, "message ID"="Update UI", "queue in"=w395) -> ("error out"=w393:errorcluster)  [unwired: 7 in, 1 out]
          }
          frame True {
          }
        }
      }
      frame "View Target Info" {
        # "Display additional information about the selected RT target in a popup window"
        n244 = Unbundle By Name(w406) -> ("Targets Information"=w405:T10[], "Filtered Targets"=w403:i32[])
        n245 = Decimal String To Number(string=w404) -> (number=w402:i32)  [unwired: 3 out]
        n246 = Index Array(array=w403, index=w402) -> (element=w401:i32)
        n247 = Index Array(array=w405, index=w401) -> (element=w397:T10)
        n248 = call "rad_Get Target Info (IP).vi"("error in (no error)"=w399, "Target settings in"=w397) -> ("error out"=w398:errorcluster, "Target settings out"=w400:T10)  [unwired: 8 in]
        n249 = case shown="No Error" w398 {
          selector: w398 -> [_ w408]
          tunnel: w400 -> [w407 _]
          frame No Error {
            n250 = call "rad_Target Info Dialog.vi"("Target Information"=w407) -> ()  [unwired: 11 out]
          }
          frame Error {
            n251 = call <vilib>:"General Error Handler.vi"("error in (no error)"=w408) -> ()  [unwired: 10 in, 5 out]
          }
        }
      }
      frame "Delete Target" {
        n252 = Unbundle By Name(w424) -> ("Targets Information"=w423:T10[], "Filtered Targets"=w411:i32[], "User Added Targets"=w412:string[])
        n253 = Decimal String To Number(string=w428) -> (number=w414:i32)  [unwired: 2 in, 1 out]
        n254 = Index Array(array=w411, index=w414) -> (element=w413:i32)
        n255 = Delete From Array(array=w423, length=1, index=w413) -> (deleted portion=w421:T10[], array with subset deleted=w422:T10[])
        n256 = Index Array(array=w421) -> (element=w420:T10)  [unwired: 1 in]
        n257 = Unbundle By Name(w420) -> ("Primary NIC.IP address"=w410:string)
        n258 = Search 1D Array(1D array=w412, element=w410) -> (index of element=w427:i32)  [unwired: 1 in]
        n259 = call "Enqueue Message with Data.vi"("error in (no error)"=w417, "message ID"="Update UI" ("Message Name"), "queue in"=w418) -> ("error out"=w416:errorcluster)  [unwired: 7 in, 1 out]
        n260 = Delete From Array(array=w412, length=1, index=w427) -> (array with subset deleted=w409:string[])  [unwired: 1 out]
        n261 = Bundle By Name(cluster=w424, "Targets Information"=w422, "User Added Targets"=w409) -> (w419:T8)
      }
      frame "**** Image Messages ****" {
      }
      frame "Refresh AppImages" {
        # "Update list of application images available in the configured folder"
        n262 = Unbundle By Name(w436) -> ("App Images Settings.App Images Temp Folder"=w437:path, "App Images Settings.App Images Folder"=w441:path)
        n263 = call "Util_Progress Show Progress Popup.vi"("Title"="Refreshing App Images", "Message"="Refreshing application images list...") -> ("error out"=w440:errorcluster)  [unwired: 2 in, 7 out]
        n264 = call "rad_List Application Images.vi"("App Image Temp Folder"=w437, "error in (no error)"=w440, "App Images Folder"=w441) -> ("error out"=w439:errorcluster, "Application Images Infomration"=w438:T13[])  [unwired: 1 in, 6 out]
        n265 = Bundle By Name(cluster=w436, "App Images Information"=w438) -> (w432:T8)
        n266 = call "Util_Progress Close Progress Popup.vi"("error in (no error)"=w439) -> ()  [unwired: 2 in, 9 out]
        n267 = call "Enqueue Message with Data.vi"("error in (no error)"=w433, "message ID"="Update UI" ("Message"), "queue in"=w434) -> ("error out"=w435:errorcluster)  [unwired: 7 in, 1 out]
      }
      frame "Configure App Image" {
        # "Update additional information (name, verison, description)\nstored with the selected application image"
        n268 = Unbundle By Name(w454) -> ("App Images Settings.App Images Temp Folder"=w450:path, "App Images Information"=w456:T13[])
        n269 = Decimal String To Number(string=w457) -> (number=w452:i32)  [unwired: 3 out]
        n270 = Index Array(array=w456, index=w452) -> (element=w451:T13)
        n271 = call "rad_Configure Application Image.vi"("Temp Folder"=w450, "error in (no error)"=w449, "App Images Information"=w451) -> ("error out"=w446:errorcluster, "Cancelled"=w444:bool, "App Images Information"=w445:T13)  [unwired: 6 in]
        n272 = Replace Array Subset(array=w456, new element=w445, index=w452) -> (w455:T13[])
        n273 = case shown="False" w444 {
          tunnel: [w461 w462] -> w448
          tunnel: w447 -> [w459 _]
          tunnel: w446 -> [w458 w462]
          frame False {
            n274 = call "Enqueue Message with Data.vi"("error in (no error)"=w458, "message ID"="Refresh AppImages", "queue in"=w459) -> ("error out"=w461:errorcluster)  [unwired: 7 in, 1 out]
          }
          frame True {
          }
        }
        n275 = Bundle By Name(cluster=w454, "App Images Information"=w455) -> (w453:T8)
      }
      frame "Configure AppImages Settings" {
        # "Update the selection of the folder where application images are stored"
        n276 = Unbundle By Name(w467) -> ("App Images Settings"=w466:T12)
        n277 = call "rad_Configure App Images Settings Dialog.vi"("App Images Settings"=w466) -> ("Cancelled"=w463:bool, "App Images Settings"=w465:T12)  [unwired: 1 in, 8 out]
        n278 = case shown="False" w463 {
          tunnel: w470 -> [w474 _]
          tunnel: w469 -> [w472 w475]
          tunnel: [w471 w475] -> w464
          frame False {
            n279 = call "Enqueue Message with Data.vi"("error in (no error)"=w472, "message ID"="Refresh AppImages", "queue in"=w474) -> ("error out"=w471:errorcluster)  [unwired: 7 in, 1 out]
          }
          frame True {
          }
        }
        n280 = Bundle By Name(cluster=w467, "App Images Settings"=w465) -> (w468:T8)
      }
      frame "View App Image Info" {
        n281 = Unbundle By Name(w480) -> ("App Images Information"=w479:T13[])
        n282 = Decimal String To Number(string=w477) -> (number=w476:i32)  [unwired: 2 in, 1 out]
        n283 = Index Array(array=w479, index=w476) -> (element=w478:T13)
        n284 = call "rad_View App Image Info.vi"("App Images Information"=w478) -> ()  [unwired: 11 in]
      }
      frame "Compare App Image" {
        n285 = Scan From String(format string="%[^(]", input string=w484) -> (remaining string=w483:string, output 1=w485:string)  [unwired: 2 in, 3 out]
        n286 = case shown="\"Image Target Compare\"" w485 {
          tunnel: w488 -> [w500 w529 w535]
          tunnel: w487 -> [w497 w521 w540]
          tunnel: w483 -> [w499 w531 _]
          tunnel: [w492 w519 w539] -> w482
          frame "Image Target Compare" {
            n287 = Unbundle By Name(w500) -> ("App Images Settings.App Images Folder"=w491:path, "App Images Settings.App Images Temp Folder"=w495:path, "App Images Information"=w505:T13[], "Targets Information"=w501:T10[], "Filtered Targets"=w502:i32[])
            n288 = Scan From String(format string="(%[^)]):%d", input string=w499, error in=w497) -> (error out=w493:errorcluster, output 1=w504:string, output 2=w506:i32)  [unwired: 1 in, 4 out]
            n289 = while {
              shift-right: [w514] -> _
              shift-left: w504 -> [w516]
              tunnel: w502 -> [w511]
              tunnel: w501 -> [w509]
              tunnel: [w508] -> w498 mode=indexing
              stop <- w513 stop-if-true
              n290 = Scan From String(format string="%d,", input string=w516) -> (remaining string=w514:string, output 1=w510:i32)  [unwired: 2 in, 3 out]
              n291 = Index Array(array=w511, index=w510) -> (element=w512:i32)
              n292 = Empty String/Path?(string/path=w514) -> (empty?=w513:bool)
              n293 = Index Array(array=w509, index=w512) -> (element=w508:T10)
            }
            n294 = Index Array(array=w505, index=w506) -> (element=w503:T13)
            n295 = Index Array(array=w498) -> (element=w489:T10)  [unwired: 1 in]
            n296 = Unbundle By Name(w503) -> ("AppImage Path"=w496:path)
            n297 = call "rad_RT Image Compare Dialog.vi"("App Images Repository"=w491, "Begin Automatically? (F)"=TRUE ("Show Front Panel?"), "Temp Folder"=w495, "error in (no error)"=w493, "Operation"=rad_Comparison_Modes."Compare Local Image With Controller", "Target settings"=w489, "Original Image Path"=w496) -> ("error out"=w492:errorcluster)  [unwired: 4 in]
          }
          frame "Only Image Selected" {
            n298 = Unbundle By Name(w529) -> ("App Images Settings.App Images Folder"=w518:path, "App Images Settings.App Images Temp Folder"=w524:path, "App Images Information"=w528:T13[])
            n299 = Scan From String(format string="(%d", input string=w531, error in=w521) -> (error out=w520:errorcluster, output 1=w527:i32)  [unwired: 1 in, 3 out]
            n300 = Index Array(array=w528, index=w527) -> (element=w526:T13)
            n301 = Unbundle By Name(w526) -> ("AppImage Path"=w525:path)
            n302 = call "rad_RT Image Compare Dialog.vi"("App Images Repository"=w518, "Begin Automatically? (F)"=FALSE ("Operate Headlessly?"), "Temp Folder"=w524, "error in (no error)"=w520, "Operation"=rad_Comparison_Modes."Compare Local Image With Controller", "Target settings"=T10 {"Hostname"="", "Serial number"="", "Product name"="", "Product code"=0, "System status"="", "Credential type"=enum."None/Unlocked", "User added?"=FALSE, "Primary NIC"={"MAC address"="", "IP Address Request Mode"=0, "IP address"="", "Subnet mask"="", "Gateway"="", "DNS server"=""}}, "Original Image Path"=w525) -> ("error out"=w519:errorcluster)  [unwired: 4 in]
          }
          frame "Generic Compare", Default {
            n303 = Unbundle By Name(w535) -> ("App Images Settings.App Images Folder"=w533:path, "App Images Settings.App Images Temp Folder"=w534:path)
            n304 = call "rad_RT Image Compare Dialog.vi"("App Images Repository"=w533, "Begin Automatically? (F)"=FALSE ("Operate Headlessly?"), "Temp Folder"=w534, "error in (no error)"=w540, "Operation"=rad_Comparison_Modes."Compare Local Image With Controller", "Target settings"=T10 {"Hostname"="", "Serial number"="", "Product name"="", "Product code"=0, "System status"="", "Credential type"=enum."None/Unlocked", "User added?"=FALSE, "Primary NIC"={"MAC address"="", "IP Address Request Mode"=0, "IP address"="", "Subnet mask"="", "Gateway"="", "DNS server"=""}}, "Original Image Path"=path "") -> ("error out"=w539:errorcluster)  [unwired: 4 in]
          }
        }
      }
      frame "Delete App Image" {
        n305 = Unbundle By Name(w557) -> ("App Images Information"=w556:T13[])
        n306 = Decimal String To Number(string=w555) -> (number=w554:i32)  [unwired: 2 in, 1 out]
        n307 = Index Array(array=w556, index=w554) -> (element=w553:T13)
        n308 = Unbundle By Name(w553) -> ("AppImage Path"=w548:path, "AppImage Properties.Name"=w550:string, "AppImage Properties.Version"=w541:string)
        n309 = Concatenate Strings("Are you sure you want to delete " ("string"), w550, " version " ("string"), w541, "?" ("string")) -> (w549:string)
        n310 = Two Button Dialog(message=w549, 2:"Delete" ("button name (\"OK\")")) -> (T button?=w547:bool)  [unwired: 1 in]
        n311 = case shown="True" w547 {
          tunnel: w548 -> [_ w564]
          tunnel: w546 -> [w558 w563]
          tunnel: [w558 w561] -> w545
          tunnel: w544 -> [_ w560]
          frame False {
          }
          frame True {
            n312 = Delete(path (use dialog)=w564, error in=w563) -> (error out=w562:errorcluster)  [unwired: 3 in, 2 out]
            n313 = call "Enqueue Message with Data.vi"("error in (no error)"=w562, "message ID"="Refresh AppImages" ("Message Name"), "queue in"=w560) -> ("error out"=w561:errorcluster)  [unwired: 7 in, 1 out]
          }
        }
      }
      frame "Retrieve AppImage" {
        # "Retrieve the application image\nfrom the selected RT target."
        n314 = Unbundle By Name(w573) -> ("App Images Settings.App Images Temp Folder"=w575:path, "App Images Settings.App Images Folder"=w569:path, "Targets Information"=w565:T10[], "Filtered Targets"=w566:i32[])
        n315 = Decimal String To Number(string=w581) -> (number=w580:i32)  [unwired: 3 out]
        n316 = Index Array(array=w566, index=w580) -> (element=w582:i32)
        n317 = Index Array(array=w565, index=w582) -> (element=w567:T10)
        n318 = call "rad_Retrieve Application Image From Target.vi"("App Images Temp Folder"=w575, "error in (no error)"=w579, "Target settings"=w567, "App Images Folder"=w569) -> ("error out"=w578:errorcluster, "Cancelled"=w570:bool, "New App Image Path"=w574:path)  [unwired: 3 in, 2 out]
        n319 = Strip Path(path=w574) -> (stripped path=w571:path)  [unwired: 1 out]
        n320 = case shown="False" w570 {
          tunnel: w578 -> [w586 w587]
          tunnel: [w585 w587] -> w577
          tunnel: w576 -> [w584 _]
          frame False {
            n321 = call "Enqueue Message with Data.vi"("error in (no error)"=w586, "message ID"="Refresh AppImages" ("Message Name"), "queue in"=w584) -> ("error out"=w585:errorcluster)  [unwired: 7 in, 1 out]
          }
          frame True {
          }
        }
        n322 = Select(t=w569, s=w570, f=w571) -> (s? t:f=w568:path)
        n323 = Bundle By Name(cluster=w573, "App Images Settings.App Images Folder"=w568) -> (w572:T8)
      }
      frame "Deploy AppImage" {
        # "Deploy the selected application image to the select RT target(s)"
        n324 = Unbundle By Name(w604) -> ("App Images Settings.App Images Temp Folder"=w594:path, "App Images Information"=w600:T13[], "Targets Information"=w596:T10[], "Filtered Targets"=w597:i32[])
        n325 = Scan From String(format string="(%[^)]):%d", input string=w603) -> (output 1=w599:string, output 2=w601:i32)  [unwired: 2 in, 5 out]
        n326 = while {
          shift-right: [w616] -> _
          shift-left: w599 -> [w618]
          tunnel: w597 -> [w613]
          tunnel: w596 -> [w611]
          tunnel: [w610] -> w593 mode=indexing
          stop <- w615 stop-if-true
          n327 = Scan From String(format string="%d,", input string=w618) -> (remaining string=w616:string, output 1=w612:i32)  [unwired: 2 in, 3 out]
          n328 = Index Array(array=w613, index=w612) -> (element=w614:i32)
          n329 = Empty String/Path?(string/path=w616) -> (empty?=w615:bool)
          n330 = Index Array(array=w611, index=w614) -> (element=w610:T10)
        }
        n331 = Index Array(array=w600, index=w601) -> (element=w598:T13)
        n332 = Unbundle By Name(w598) -> ("AppImage Path"=w595:path)
        n333 = call "rad_Deploy Application Image.vi"("App Image Temp Folder"=w594, "error in (no error)"=w592, "Selected Targets"=w593, "App Image Path"=w595) -> ("error out"=w590:errorcluster, "Cancelled"=w588:bool)  [unwired: 6 out]
        n334 = case shown="False" w588 {
          tunnel: [w608 w609] -> w591
          tunnel: w590 -> [w607 w609]
          tunnel: w589 -> [w605 _]
          frame False {
            n335 = call "Enqueue Message with Data.vi"("error in (no error)"=w607, "message ID"="Refresh Targets" ("Message Name"), "queue in"=w605) -> ("error out"=w608:errorcluster)  [unwired: 7 in, 1 out]
          }
          frame True {
          }
        }
      }
      frame "Convert Images" {
        n336 = Unbundle By Name(w620) -> ("App Images Settings.App Images Folder"=w619:path)
        n337 = call "Util_ConvertImageToLatest.vi"("error in (no error)"=w625, "Image Path"=w619) -> ("error out"=w623:errorcluster)  [unwired: 9 in]
        n338 = call "Enqueue Message with Data.vi"("error in (no error)"=w623, "message ID"="Refresh AppImages" ("Message Name"), "queue in"=w621) -> ("error out"=w622:errorcluster)  [unwired: 7 in, 1 out]
      }
    }
    n339 = local write "State"(w164) -> ()
  }
  n340 = call "Resize Front Panel Main.vi"("Left Listbox"=w26, "Top Level VI"=w27, "Stop"=w28, "Number of Columns"=4, "Right Listbox"=w25, "Left Splitter"=w24, "Right Splitter"=w23, "Left Pane Items"=w17, "Mid Pane Items"=w13, "Right Pane Items"=w8) -> ()  [unwired: 5 in, 1 out]
  n341 = local write "Exit"(w7) -> ()
